vi "TDS Comms Read Data.vi"(8 "error in (no error)":errorcluster, 10 "Read Settings":string, 11 "Address":string) -> (0 "error out":errorcluster, 2 "Successful?":bool, 3 "Read Data":string)   [LabVIEW 2025, in "Interface Functions.lvlib"]
uses:
  Interface Functions.lvlib
panel:
  # "Comms Read Data"
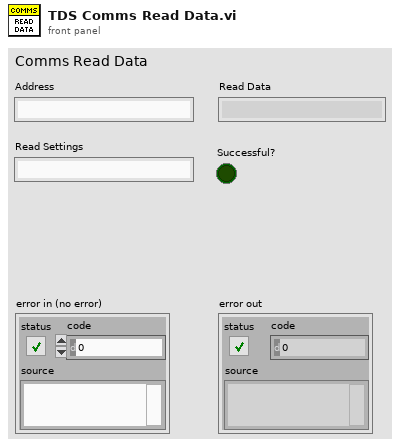
[diagram p1: front panel]
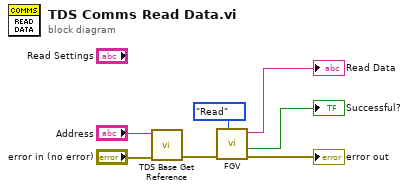
[diagram p0: block diagram]
diagram:
  n1 = call "TDS Base Get Reference.vi"("error in (no error)"="error in (no error)", "Address"="Address") -> ("error out"=w5:errorcluster)  [unwired: 8 in, 1 out]
  n2 = call "FGV.vi"("Action"=enum16{"Initialize", "Read", "Write"}."Read", "error in (no error)"=w5) -> ("error out"=→"error out":errorcluster, "Successful"=→"Successful?":bool, "Read Data"=→"Read Data":string)  [unwired: 7 in]
